vi "Transient SA.vi"() -> ()   [LabVIEW 2015]
uses:
  <vilib>/Platform/TimedLoop/XDataNode/timing_clust.ctl
  <vilib>/Platform/TimedLoop/XDataNode/nitl_modes.ctl
  <vilib>/Platform/TimedLoop/XDataNode/wakeup.ctl
  <vilib>/DAQmx/read.llb/DAQmx Read (Analog DBL 1Chan 1Samp).vi
  <vilib>/DAQmx/read.llb/DAQmx Read (Analog 1D DBL NChan 1Samp).vi
  <vilib>/DAQmx/create/channels.llb/DAQmx Create Channel (AI-Voltage-Basic).vi
  <vilib>/DAQmx/miscellaneous.llb/DAQmx Fill In Error Info.vi
  <vilib>/Platform/TimedLoop/XDataNode/XDataNode.xnode
  Program Files/neMESYS_SDK/neMESYS LabVIEW Kit/neMESYS LabVIEW Integration Kit.lvlib
  <vilib>/Platform/TimedLoop/XDataNode/XDNodeRunTimeDep.lvlib
  Conor/Temp CN7500/Omega CN7500/Omega CN7500.lvlib
panel:
  out "Iteration Number":dbl
  in  "Ramp Temp":bool
  in  "Temp Decrease per Minute":dbl
  in  "Start Temp":dbl
  in  "Minutes at Start Conditions":dbl
  in  "Ramp Flow":bool
  in  "Flow Decrease per Minute":dbl
  in  "Start Flowrate":dbl
  in  "Flowrate 4":dbl
  in  "Flowrate 3":dbl
  in  "Flowrate 2":dbl
  in  "Flowrate 1":dbl
  in  "Temp Set Point":dbl
  out "Liquid Inlet Pressure (bar g)":dbl
  in  "Liquid P sensor Terminal Configuration":i32(ring)=-1 items=["default"=-1, "RSE"=10083, "NRSE"=10078, "Differential"=10106, "Pseudodifferential"=12529]
  in  "Liquid P sensor Physical Channel":tag="Dev1/ai0"
  in  "Safety or Emergency Syringe Control":bool
  out "Total Flowrate (uL/min)":dbl
  out "Gas Back Pressure (barg)":dbl
  in  "Shut down in empty?\nLeft off, right on":bool
  in  "Clear":bool
  out "Safety Shut Down Pressure (barg)":dbl
  out "Calculated Pressure":dbl[](graph)
  out "Safety Shut Down Temp":dbl
  out "Actual Temp (oC)":dbl
  out "Temperature":dynamicdata(graph)
  out "Temp Set Point (oC)":dbl
  in  "Stop everything":bool
  in  "Refill 4":bool
  in  "Refill 3":bool
  in  "Refill 2":bool
  in  "Refill 1":bool
  in  "Empty 4":bool
  in  "Empty 3":bool
  in  "Empty 2":bool
  in  "Empty 1":bool
  in  "Calibrate 4":bool
  in  "Calibrate 3":bool
  in  "Calibrate 2":bool
  in  "Calibrate 1":bool
  in  "Stop Dose 4":bool
  in  "Stop Dose 3":bool
  in  "Stop Dose 2":bool
  in  "Stop Dose 1":bool
  out "Syringe Level 4":dbl(slide) scale=0.0..5500.0
  out "Syringe Level 3":dbl(slide) scale=0.0..5500.0
  out "Syringe Level 2":dbl(slide) scale=0.0..5500.0
  out "Syringe Level 1":dbl(slide) scale=0.0..5500.0
  out "Flowrate 4 Ethanol":dbl
  out "Flowrate 3 Acid":dbl
  out "Flowrate 2 High":dbl
  out "Flowrate 1 Low":dbl
  # "Safety (start and end)"
  # "Current Conditions"
  # "(uL/min)"
  # "Coerced to nearest possible"
  # "If either ramps are off you need to manually enter the constant flowrate or temperature in the \nbottom sections"
  # "This code just uses 2 syringes\nThe ones at the right hand side"
  # "Emergency Syringe Control Below"
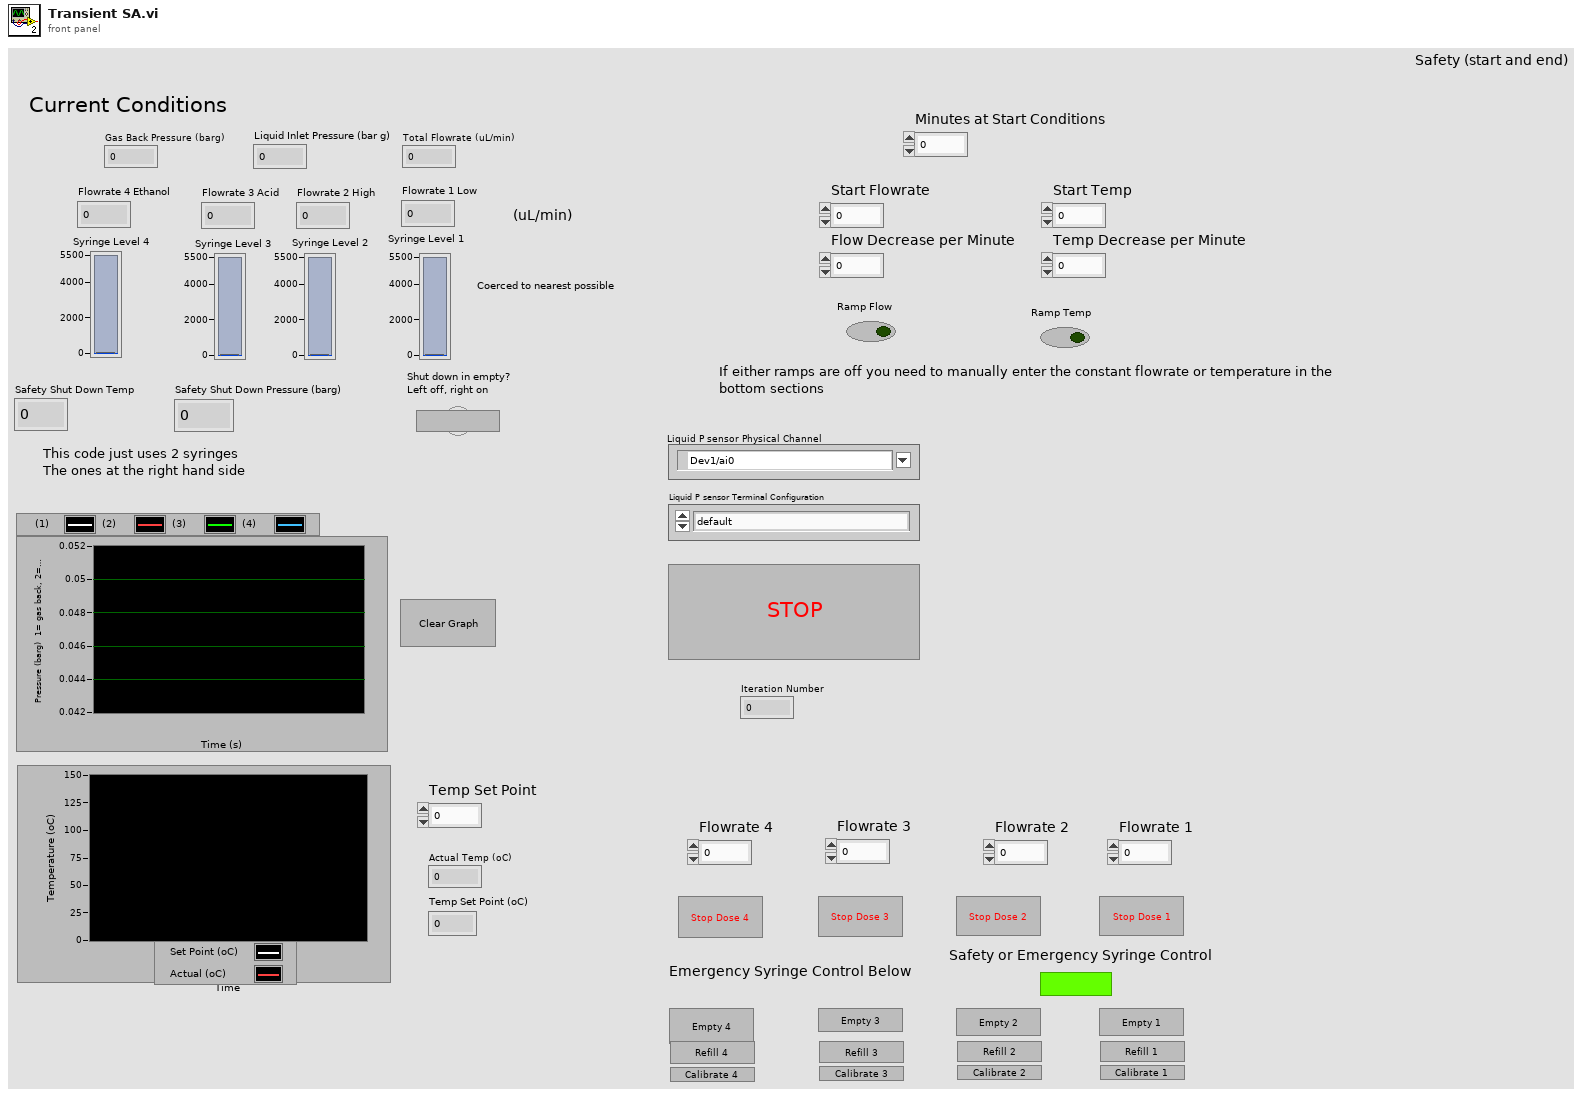
[diagram p1: front panel]
types:
  T1 = typedef "XDNodeRunTimeDep.lvlib/timing_clust.ctl" = cluster{"Expected End [f-1]":u64, "Actual End [f-1]":u64, "Finished Late? [f-1]":bool, "Expected End [i-1]":u64, "Actual End [i-1]":u64, "Finished Late? [i-1]":bool, "Expected Start [i]":u64, "Actual Start [i]":u64, "Expected Start [f]":u64, "Actual Start [f]":u64, "Source Name":string, "Structure Name":string, "Period":i64, "Deadline":i64, "Offset":i64, "Start":i64, "Priority":i32, "Timeout":i32, "Mode":T2, "Wakeup Reason":T3, "Error":errorcluster, "Source Type":string, "Secondary Source Type":string, "Global End Time":u64, "Global Start Time":u64, "Frame Duration":u64, "Iteration Duration":u64, "Assigned CPU":i32, "I/O Scan Engine Mode":u32}
  T2 = typedef "XDNodeRunTimeDep.lvlib/nitl_modes.ctl" = enum32{"No Change", "Process missed periods, maintain original phase", "Discard missed periods, maintain original phase", "Process missed periods, ignore original phase", "Discard missed periods, ignore original phase"}
  T3 = typedef "XDNodeRunTimeDep.lvlib/wakeup.ctl" = enum32{"Normal", "Aborted", "Asynchronous wakeup", "Timing source error", "Timed loop error", "Timeout"}
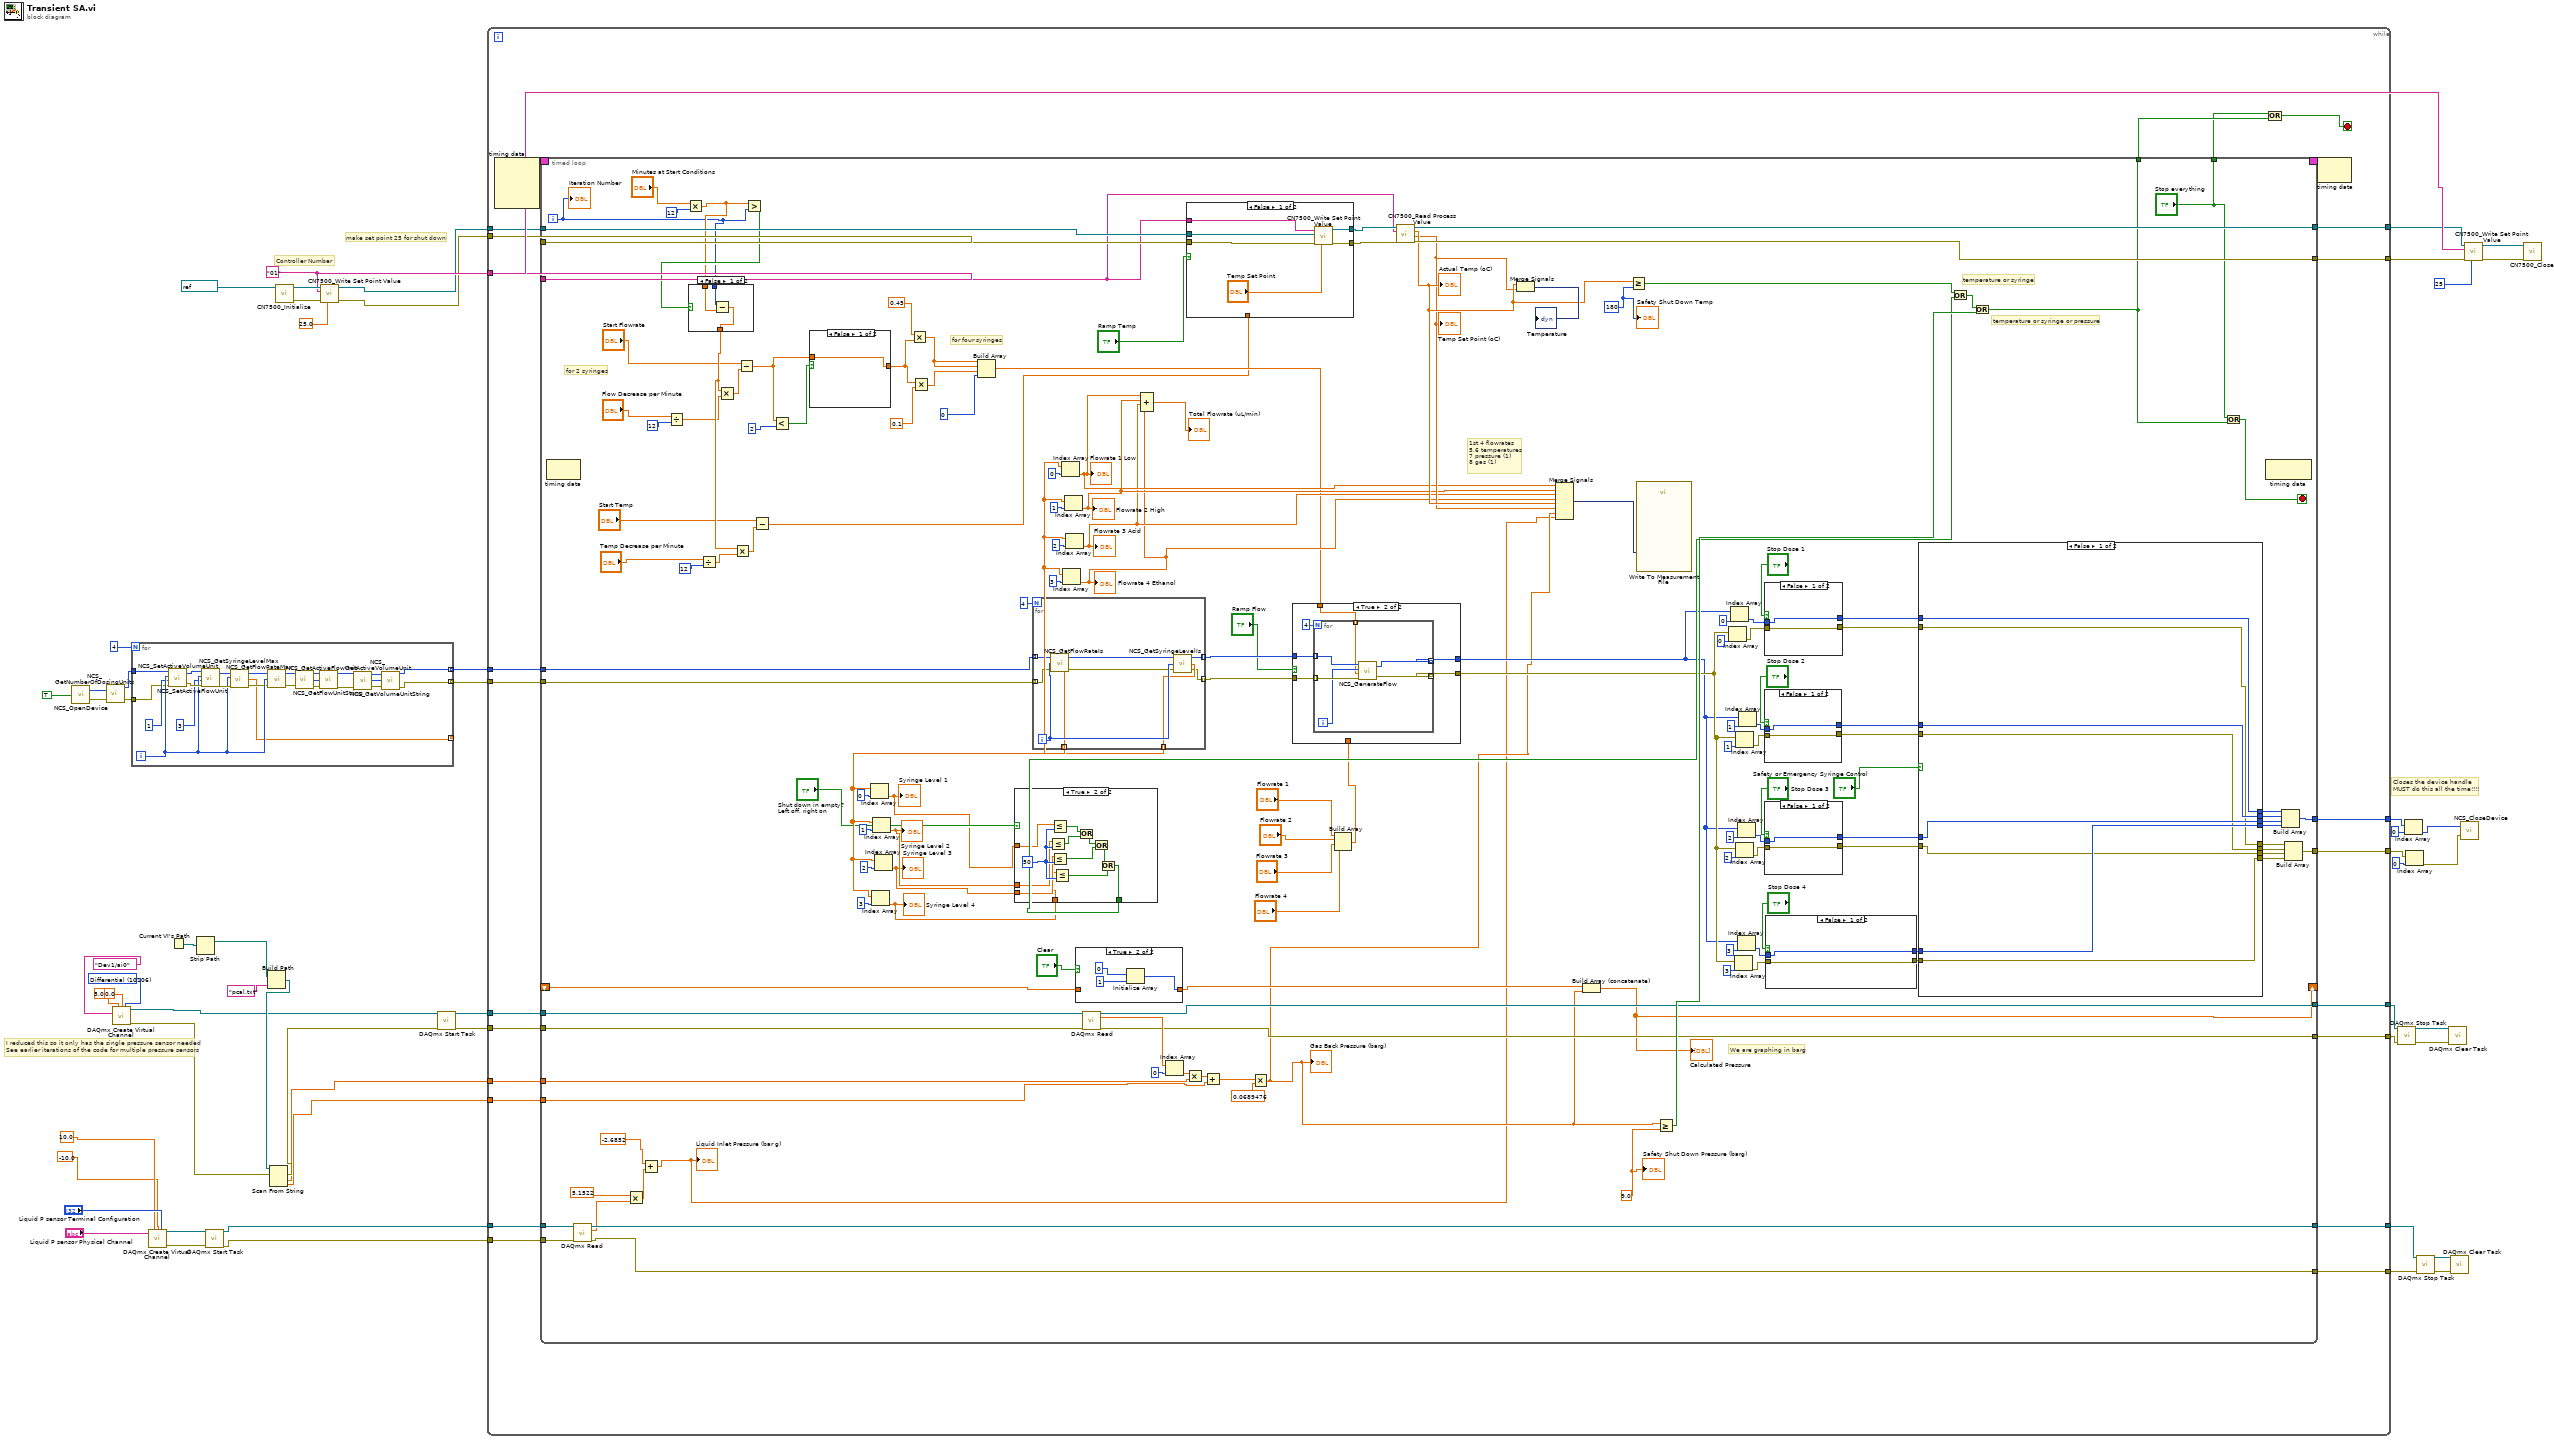
[diagram p0: block diagram]
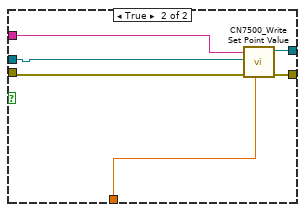
[diagram p2: hidden frame]
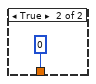
[diagram p3: hidden frame]
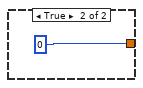
[diagram p4: hidden frame]
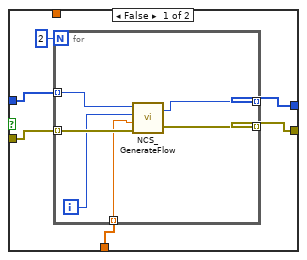
[diagram p5: hidden frame]
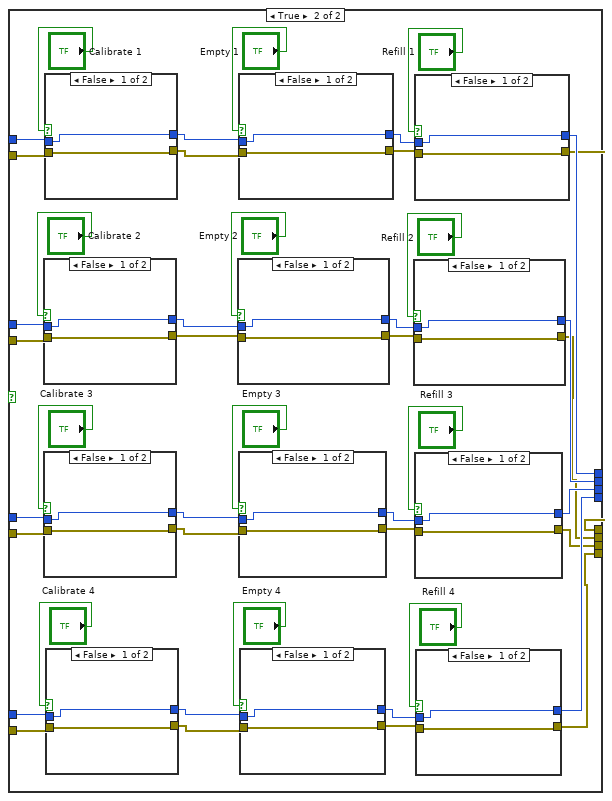
[diagram p6: hidden frame]
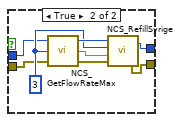
[diagram p7: hidden frame]
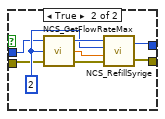
[diagram p8: hidden frame]
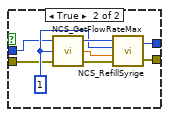
[diagram p9: hidden frame]
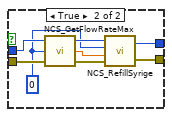
[diagram p10: hidden frame]
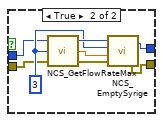
[diagram p11: hidden frame]
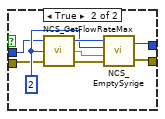
[diagram p12: hidden frame]
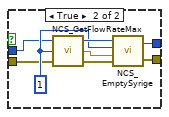
[diagram p13: hidden frame]
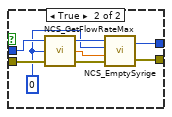
[diagram p14: hidden frame]
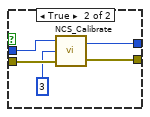
[diagram p15: hidden frame]
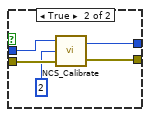
[diagram p16: hidden frame]
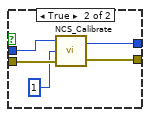
[diagram p17: hidden frame]
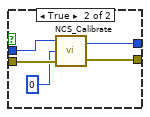
[diagram p18: hidden frame]
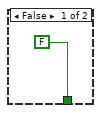
[diagram p19: hidden frame]
diagram:
  w29 = 10106 items=["default"=-1, "RSE"=10083, "NRSE"=10078, "Differential"=10106, "Pseudodifferential"=12529] ("input terminal configuration")
  w36 = "01" ("Controller Number")
  # "I reduced this so it only has the single pressure sensor needed\nSee earlier iterations of the code for multiple pressure sensors"
  # "make set point 25 for shut down"
  # "Controller Number"
  # "Closes the device handle \nMUST do this all the time!!!!"
  n1 = call "NCS_OpenDevice.vi"("show status window"=TRUE) -> ("device handle"=w55:u32, "error out"=w54:errorcluster)
  n2 = call "NCS_GetNumberOfDosingUnits.vi"("device handle in"=w55, "error in (no error)"=w54) -> ("device handle out"=w52:u32, "error out"=w53:errorcluster)  [unwired: 1 out]
  n3 = call-poly <vilib>:"DAQmx Create Virtual Channel.vi"("maximum value"=5.0, "minimum value"=0.0, "input terminal configuration"=w29, "physical channels"=tag "Dev1/ai0") -> ("task out"=w13:refnum<k21>, "error out"=w14:errorcluster)  [unwired: 10 in]
  n4 = for {
    N: 4 -> [_]
    tunnel: [w61] -> w51 mode=indexing
    tunnel: [w60] -> w50 mode=indexing
    tunnel: [w74] -> _ mode=indexing
    tunnel: w53 -> [w59]
    tunnel: w52 -> [w58]
    i -> [w77]
    n5 = call "NCS_SetActiveVolumeUnit.vi"("error in (no error)"=w59, "active volume unit"=1, "dosingunit"=w77, "device handle in"=w58) -> ("error out"=w80:errorcluster, "device handle out"=w81:u32)
    n6 = call "NCS_SetActiveFlowUnit.vi"("error in (no error)"=w80, "active flow unit"=3, "dosingunit"=w77, "device handle in"=w81) -> ("error out"=w78:errorcluster, "device handle out"=w79:u32)
    n7 = call "NCS_GetSyringeLevelMax.vi"("error in (no error)"=w78, "dosingunit"=w77, "device handle in"=w79) -> ("error out"=w75:errorcluster, "syringe level max"=w74:dbl, "device handle out"=w76:u32)  [unwired: 1 out]
    n8 = call "NCS_GetFlowRateMax.vi"("error in (no error)"=w75, "dosingunit"=w77, "device handle in"=w76) -> ("error out"=w62:errorcluster, "device handle out"=w63:u32)  [unwired: 1 out]
    n9 = call "NCS_GetActiveFlowUnit.vi"("error in (no error)"=w62, "device handle in"=w63) -> ("error out"=w70:errorcluster, "active flow unit"=w69:u8, "device handle out"=w71:u32)  [unwired: 1 in]
    n10 = call "NCS_GetFlowUnitString.vi"("device handle in"=w71, "flow unit id"=w69, "error in (no error)"=w70) -> ("device handle out"=w66:u32, "error out"=w65:errorcluster)  [unwired: 2 out]
    n11 = call "NCS_GetActiveVolumeUnit.vi"("error in (no error)"=w65, "device handle in"=w66) -> ("error out"=w67:errorcluster, "active volume unit"=w68:u8, "device handle out"=w64:u32)  [unwired: 1 in]
    n12 = call "NCS_GetVolumeUnitString.vi"("device handle in"=w64, "volume unit id"=w68, "error in (no error)"=w67) -> ("device handle out"=w61:u32, "error out"=w60:errorcluster)  [unwired: 2 out]
  }
  n13 = call-poly <vilib>:"DAQmx Create Virtual Channel.vi"("maximum value"=10.0, "minimum value"=-10.0 ("maximum value"), "input terminal configuration"="Liquid P sensor Terminal Configuration", "physical channels"="Liquid P sensor Physical Channel") -> ("task out"=w9:refnum<k21>, "error out"=w10:errorcluster)  [unwired: 10 in]
  n14 = Current VI's Path() -> (path=w27:path)
  n15 = Strip Path(path=w27) -> (stripped path=w25:path)  [unwired: 1 out]
  n16 = call <vilib>:"DAQmx Start Task.vi"("task/channels in"=w9, "error in"=w10) -> ("task out"=w8:refnum<k21>, "error out"=w7:errorcluster)  [unwired: 12 in]
  n17 = Build Path(base path=w25, name or relative path="pcal.txt") -> (appended path=w26:path)
  n18 = Scan From String(w26, w14) -> (w23:errorcluster, output 1=w20:dbl, output 2=w19:dbl)  [unwired: 3 in, 1 out]
  n19 = call "CN7500_Initialize.vi"("VISA resource name"=refnum<visa-resource-name> "COM8") -> ("error out"=w42:errorcluster, "VISA resource name out"=w43:refnum<visa-resource-name>)  [unwired: 9 in]
  n20 = call "CN7500_Write Set Point Value.vi"("Target Set Point Value"=25.0, "error in (no error)"=w42, "Controller Number"=w36, "VISA In"=w43) -> ("error out"=w34:errorcluster, "VISA Out"=w35:refnum<visa-resource-name>)  [unwired: 6 in]
  n21 = call <vilib>:"DAQmx Start Task.vi"("task/channels in"=w13, "error in"=w23) -> ("task out"=w22:refnum<k21>, "error out"=w21:errorcluster)  [unwired: 12 in]
  n22 = while {
    tunnel: w51 -> [w105]
    tunnel: w50 -> [w104]
    tunnel: [w103] -> w45
    tunnel: [w102] -> w44
    tunnel: w36 -> [w99]
    tunnel: w35 -> [w98]
    tunnel: w34 -> [w97]
    tunnel: [w96] -> w33
    tunnel: [w95] -> w32
    tunnel: w22 -> [w93]
    tunnel: w21 -> [w92]
    tunnel: w20 -> [w91]
    tunnel: w19 -> [w90]
    tunnel: [w89] -> w16
    tunnel: [w88] -> w15
    tunnel: w8 -> [w85]
    tunnel: w7 -> [w84]
    tunnel: [w83] -> w5
    tunnel: [w82] -> w3
    stop <- w87 stop-if-true
    n23 = node-c288() -> (w101:T1)  [unwired: 4 in]
    n24 = timed-loop {
      tunnel: w105 -> [w250]
      tunnel: w104 -> [w249]
      tunnel: [w200] -> w103
      tunnel: [w199] -> w102
      timing: w101 -> [_]
      timing-out: [_] -> w100
      tunnel: w99 -> [w193]
      tunnel: w98 -> [w197]
      tunnel: w97 -> [w196]
      tunnel: [w192] -> w96
      tunnel: [w191] -> w95
      tunnel: [w135] -> w94
      tunnel: w93 -> [w179]
      tunnel: w92 -> [w178]
      tunnel: w91 -> [w177]
      tunnel: w90 -> [w176]
      shift-right: [w156] -> _
      shift-left: _ -> [w169]
      tunnel: [w172] -> w89
      tunnel: [w171] -> w88
      tunnel: ["Stop everything"] -> w86
      tunnel: w85 -> [w155]
      tunnel: w84 -> [w154]
      tunnel: [w153] -> w83
      tunnel: [w152] -> w82
      i -> [w114]
      stop <- w167 stop-if-true
      w175 = 9.0 ("Safety Shut Down Pressure (barg)")
      w189 = 180
      # "for four syringes"
      # "for 2 syringes"
      # "1st 4 flowrates\n5,6 temperatures\n7 pressure (1)\n8 gas (1)"
      # "temperature or syringe or pressure"
      # "We are graphing in barg"
      # "temperature or syringe"
      n25 = node-c288() -> ()  [unwired: 1 in, 1 out]
      n26 = call-poly <vilib>:"DAQmx Read.vi"("task/channels in"=w155, "error in"=w154) -> ("task out"=w153:refnum<k21>, "data"=w148:dbl, "error out"=w152:errorcluster)  [unwired: 11 in]
      n27 = Multiply(x=5.1522, y=w148) -> (x*y=w151:dbl)
      n28 = Add(x=-2.6852, y=w151) -> (x+y=w146:dbl)
      "Liquid Inlet Pressure (bar g)" <- w146
      n29 = Divide(x="Flow Decrease per Minute", y=12) -> (x/y=w112:dbl)
      n30 = Multiply(x="Minutes at Start Conditions", y=12) -> (x*y=w123:dbl)
      n31 = Divide(x="Temp Decrease per Minute", y=12) -> (x/y=w119:dbl)
      n32 = Greater?(x=w123, y=w114) -> (0:w124:bool)
      n33 = case shown="False" w124 {
        tunnel: [w264 0] -> w118
        tunnel: w114 -> [w266 _]
        tunnel: w123 -> [w265 _]
        frame False {
          n34 = Subtract(x=w266, y=w265) -> (x-y=w264:dbl)
        }
        frame True {
        }
      }
      n35 = Multiply(x=w118, y=w112) -> (x*y=w132:dbl)
      n36 = Multiply(x=w118, y=w119) -> (x*y=w120:dbl)
      n37 = Subtract(x="Start Flowrate", y=w132) -> (x-y=w127:dbl)
      n38 = Subtract(x="Start Temp", y=w120) -> (x-y=w115:dbl)
      n39 = Less?(x=w127, y=2) -> (x < y?=w128:bool)
      n40 = case shown="False" w128 {
        tunnel: [w268 0] -> w108
        tunnel: w127 -> [w268 _]
        frame False {
        }
        frame True {
        }
      }
      n41 = Multiply(x=0.45, y=w108) -> (x*y=w107:dbl)
      n42 = Multiply(x=w108, y=0.1) -> (x*y=w106:dbl)
      n43 = Build Array(w107, w107, w106, 0) -> (w130:dbl[])
      n44 = for {
        N: 4 -> [_]
        tunnel: w250 -> [w509] mode=indexing
        tunnel: [w507] -> w244 mode=indexing
        tunnel: [w504] -> w239 mode=indexing
        tunnel: [w503] -> w238 mode=indexing
        tunnel: [w502] -> w237 mode=indexing
        tunnel: w249 -> [w501] mode=indexing
        i -> [w508]
        n45 = call "NCS_GetFlowRateIs.vi"("error in (no error)"=w501, "dosingunit"=w508, "device handle in"=w509) -> ("error out"=w505:errorcluster, "flowrate is"=w507:dbl, "device handle out"=w506:u32)
        n46 = call "NCS_GetSyringeLevelIs.vi"("error in (no error)"=w505, "dosingunit"=w508, "device handle in"=w506) -> ("error out"=w502:errorcluster, "syringe level is"=w504:dbl, "device handle out"=w503:u32)
      }
      n47 = Index Array(array=w239, index=0) -> (element=w164:dbl)
      "Syringe Level 1" <- w164
      n48 = Index Array(array=w239, index=3) -> (element=w161:dbl)
      "Syringe Level 4" <- w161
      n49 = Index Array(array=w239, index=1) -> (element=w163:dbl)
      "Syringe Level 2" <- w163
      n50 = Index Array(array=w239, index=2) -> (element=w162:dbl)
      "Syringe Level 3" <- w162
      n51 = case shown="True" "Shut down in empty?\nLeft off, right on" {
        tunnel: [FALSE w459] -> w165
        tunnel: w164 -> [_ w458]
        tunnel: w163 -> [_ w457]
        tunnel: w162 -> [_ w456]
        tunnel: w161 -> [_ w455]
        frame False {
        }
        frame True {
          w460 = 50
          n52 = Less Or Equal?(x=w457, y=w460) -> (x <= y?=w466:bool)
          n53 = Less Or Equal?(x=w458, y=w460) -> (x <= y?=w461:bool)
          n54 = Less Or Equal?(x=w456, y=w460) -> (x <= y?=w464:bool)
          n55 = Less Or Equal?(x=w455, y=w460) -> (x <= y?=w462:bool)
          n56 = Or(x=w461, y=w466) -> (x .or. y?=w465:bool)
          n57 = Or(x=w465, y=w464) -> (x .or. y?=w463:bool)
          n58 = Or(x=w463, y=w462) -> (x .or. y?=w459:bool)
        }
      }
      n59 = Index Array(array=w244, index=0) -> (element=w144:dbl)
      "Flowrate 1 Low" <- w144
      n60 = Index Array(array=w244, index=3) -> (element=w141:dbl)
      "Flowrate 4 Ethanol" <- w141
      n61 = Index Array(array=w244, index=1) -> (element=w143:dbl)
      "Flowrate 2 High" <- w143
      n62 = Index Array(array=w244, index=2) -> (element=w142:dbl)
      "Flowrate 3 Acid" <- w142
      n63 = case shown="True" "Clear" {
        tunnel: w169 -> [w467 _]
        tunnel: [w467 w468] -> w168
        frame False {
        }
        frame True {
          n64 = Initialize Array(0, 1) -> (w468:i32[])
        }
      }
      n65 = call-poly <vilib>:"DAQmx Read.vi"("task/channels in"=w179, "error in"=w178) -> ("task out"=w172:refnum<k21>, "data"=w184:dbl[], "error out"=w171:errorcluster)  [unwired: 11 in]
      n66 = Compound Arithmetic op=ADD(w144, w143, w142, w141) -> (→"Total Flowrate (uL/min)":dbl)
      n67 = Index Array(array=w184, index=0) -> (element=w182:dbl)
      n68 = Multiply(x=w182, y=w177) -> (x*y=w183:dbl)
      n69 = case shown="False" "Ramp Temp" {
        tunnel: w197 -> [w257 w262]
        tunnel: w196 -> [w256 w261]
        tunnel: [w255 w260] -> w195
        tunnel: [w254 w259] -> w194
        tunnel: w193 -> [w253 w263]
        tunnel: w115 -> [_ w258]
        frame False {
          n70 = call "CN7500_Write Set Point Value.vi"("Target Set Point Value"="Temp Set Point", "error in (no error)"=w256, "Controller Number"=w253, "VISA In"=w257) -> ("error out"=w254:errorcluster, "VISA Out"=w255:refnum<visa-resource-name>)  [unwired: 6 in]
        }
        frame True {
          n71 = call "CN7500_Write Set Point Value.vi"("Target Set Point Value"=w258, "error in (no error)"=w261, "Controller Number"=w263, "VISA In"=w262) -> ("error out"=w259:errorcluster, "VISA Out"=w260:refnum<visa-resource-name>)  [unwired: 6 in]
        }
      }
      n72 = Add(x=w183, y=w176) -> (x+y=w180:dbl)
      n73 = Multiply(x=w180, y=0.0689476) -> (x*y=w147:dbl)
      "Gas Back Pressure (barg)" <- w147
      n74 = Build Array("Flowrate 1", "Flowrate 2", "Flowrate 3", "Flowrate 4") -> (w136:dbl[])
      n75 = case shown="True" "Ramp Flow" {
        tunnel: w238 -> [w274 w287]
        tunnel: w237 -> [w273 w286]
        tunnel: [w271 w285] -> w159
        tunnel: [w270 w284] -> w158
        tunnel: w136 -> [w272 _]
        tunnel: w130 -> [_ w282]
        frame False {
          n76 = for {
            N: 2 -> [_]
            tunnel: w274 -> [w281] mode=indexing
            tunnel: w273 -> [w280] mode=indexing
            tunnel: [w279] -> w271 mode=indexing
            tunnel: [w278] -> w270 mode=indexing
            tunnel: w272 -> [w276] mode=indexing
            i -> [w277]
            n77 = call "NCS_GenerateFlow.vi"("error in (no error)"=w280, "flowrate"=w276, "dosingunit"=w277, "device handle in"=w281) -> ("error out"=w279:errorcluster, "device handle out"=w278:u32)
          }
        }
        frame True {
          n78 = for {
            N: 4 -> [_]
            tunnel: w287 -> [w293] mode=indexing
            tunnel: w286 -> [w292] mode=indexing
            tunnel: [w291] -> w285 mode=indexing
            tunnel: [w290] -> w284 mode=indexing
            tunnel: w282 -> [w288] mode=indexing
            i -> [w289]
            n79 = call "NCS_GenerateFlow.vi"("error in (no error)"=w292, "flowrate"=w288, "dosingunit"=w289, "device handle in"=w293) -> ("error out"=w291:errorcluster, "device handle out"=w290:u32)
          }
        }
      }
      n80 = call "CN7500_Read Process Value.vi"("error in (no error)"=w194, "Controller Number"=w193, "VISA In"=w195) -> ("error out"=w192:errorcluster, "Set Point Value"=w186:dbl, "Process Value"=w187:dbl, "VISA Out"=w191:refnum<visa-resource-name>)  [unwired: 5 in]
      "Temp Set Point (oC)" <- w186
      "Actual Temp (oC)" <- w187
      n81 = Merge Signals(w187, w186) -> (→"Temperature":dynamicdata)
      n82 = Merge Signals(w144, w143, w142, w141, w187, w186, w147, w146) -> (w198:dynamicdata)
      n83 = Build Array (concatenate)(w168, w147) -> (w156:dbl[])
      "Calculated Pressure" <- w156
      n84 = Greater Or Equal?(x=w187, y=w189) -> (x >= y?=w188:bool)
      n85 = call "Write To Measurement File"("Signals"=w198) -> ()  [unwired: 16 in, 3 out]
      n86 = Greater Or Equal?(x=w147, y=w175) -> (x >= y?=w173:bool)
      n87 = Index Array(array=w159, index=0) -> (element=w227:errorcluster)
      n88 = Index Array(array=w158, index=0) -> (element=w228:u32)
      n89 = Index Array(array=w159, index=3) -> (element=w217:errorcluster)
      n90 = Index Array(array=w159, index=2) -> (element=w219:errorcluster)
      n91 = Index Array(array=w159, index=1) -> (element=w221:errorcluster)
      n92 = Index Array(array=w158, index=3) -> (element=w218:u32)
      n93 = Index Array(array=w158, index=2) -> (element=w220:u32)
      n94 = Index Array(array=w158, index=1) -> (element=w222:u32)
      n95 = case shown="False" "Stop Dose 2" {
        tunnel: w222 -> [w488 w493]
        tunnel: w221 -> [w487 w492]
        tunnel: [w488 w491] -> w214
        tunnel: [w487 w490] -> w213
        frame False {
        }
        frame True {
          n96 = call "NCS_Stop.vi"("error in (no error)"=w492, "dosingunit"=1, "device handle in"=w493) -> ("error out"=w490:errorcluster, "device handle out"=w491:u32)
        }
      }
      n97 = case shown="False" "Stop Dose 1" {
        tunnel: w228 -> [w495 w500]
        tunnel: w227 -> [w494 w499]
        tunnel: [w495 w498] -> w216
        tunnel: [w494 w497] -> w215
        frame False {
        }
        frame True {
          n98 = call "NCS_Stop.vi"("error in (no error)"=w499, "dosingunit"=0, "device handle in"=w500) -> ("error out"=w497:errorcluster, "device handle out"=w498:u32)
        }
      }
      n99 = case shown="False" "Stop Dose 3" {
        tunnel: w220 -> [w481 w486]
        tunnel: w219 -> [w480 w485]
        tunnel: [w481 w484] -> w212
        tunnel: [w480 w483] -> w211
        frame False {
        }
        frame True {
          n100 = call "NCS_Stop.vi"("error in (no error)"=w485, "dosingunit"=2, "device handle in"=w486) -> ("error out"=w483:errorcluster, "device handle out"=w484:u32)
        }
      }
      n101 = case shown="False" "Stop Dose 4" {
        tunnel: w218 -> [w474 w479]
        tunnel: w217 -> [w473 w478]
        tunnel: [w474 w477] -> w210
        tunnel: [w473 w476] -> w209
        frame False {
        }
        frame True {
          n102 = call "NCS_Stop.vi"("error in (no error)"=w478, "dosingunit"=3, "device handle in"=w479) -> ("error out"=w476:errorcluster, "device handle out"=w477:u32)
        }
      }
      n103 = case shown="False" "Safety or Emergency Syringe Control" {
        tunnel: w216 -> [w301 w342]
        tunnel: w215 -> [w297 w341]
        tunnel: w214 -> [w300 w340]
        tunnel: w213 -> [w296 w339]
        tunnel: w212 -> [w299 w338]
        tunnel: w211 -> [w295 w337]
        tunnel: w210 -> [w298 w336]
        tunnel: w209 -> [w294 w335]
        tunnel: [w301 w312] -> w208
        tunnel: [w300 w311] -> w207
        tunnel: [w299 w310] -> w206
        tunnel: [w298 w309] -> w205
        tunnel: [w296 w308] -> w204
        tunnel: [w295 w307] -> w203
        tunnel: [w294 w306] -> w202
        tunnel: [w297 w302] -> w201
        frame False {
        }
        frame True {
          n104 = case shown="False" "Calibrate 2" {
            tunnel: w340 -> [w441 w446]
            tunnel: w339 -> [w440 w445]
            tunnel: [w441 w444] -> w329
            tunnel: [w440 w443] -> w328
            frame False {
            }
            frame True {
              n105 = call "NCS_Calibrate.vi"("error in (no error)"=w445, "dosingunit"=1, "device handle in"=w446) -> ("error out"=w443:errorcluster, "device handle out"=w444:u32)
            }
          }
          n106 = case shown="False" "Calibrate 3" {
            tunnel: w338 -> [w434 w439]
            tunnel: w337 -> [w433 w438]
            tunnel: [w434 w437] -> w327
            tunnel: [w433 w436] -> w326
            frame False {
            }
            frame True {
              n107 = call "NCS_Calibrate.vi"("error in (no error)"=w438, "dosingunit"=2, "device handle in"=w439) -> ("error out"=w436:errorcluster, "device handle out"=w437:u32)
            }
          }
          n108 = case shown="False" "Calibrate 1" {
            tunnel: w342 -> [w448 w453]
            tunnel: w341 -> [w447 w452]
            tunnel: [w448 w451] -> w331
            tunnel: [w447 w450] -> w330
            frame False {
            }
            frame True {
              n109 = call "NCS_Calibrate.vi"("error in (no error)"=w452, "dosingunit"=0, "device handle in"=w453) -> ("error out"=w450:errorcluster, "device handle out"=w451:u32)
            }
          }
          n110 = case shown="False" "Calibrate 4" {
            tunnel: w336 -> [w427 w432]
            tunnel: w335 -> [w426 w431]
            tunnel: [w427 w430] -> w325
            tunnel: [w426 w429] -> w324
            frame False {
            }
            frame True {
              n111 = call "NCS_Calibrate.vi"("error in (no error)"=w431, "dosingunit"=3, "device handle in"=w432) -> ("error out"=w429:errorcluster, "device handle out"=w430:u32)
            }
          }
          n112 = case shown="False" "Empty 2" {
            tunnel: w329 -> [w407 w411]
            tunnel: w328 -> [w406 w409]
            tunnel: [w407 w410] -> w315
            tunnel: [w406 w408] -> w316
            frame False {
            }
            frame True {
              w413 = 1
              n113 = call "NCS_GetFlowRateMax.vi"("error in (no error)"=w409, "dosingunit"=w413, "device handle in"=w411) -> ("error out"=w414:errorcluster, "flow rate max"=w412:dbl, "device handle out"=w415:u32)
              n114 = call "NCS_EmptySyrige.vi"("error in (no error)"=w414, "flowrate"=w412, "dosingunit"=w413, "device handle in"=w415) -> ("error out"=w408:errorcluster, "device handle out"=w410:u32)
            }
          }
          n115 = case shown="False" "Empty 1" {
            tunnel: w331 -> [w417 w425]
            tunnel: w330 -> [w416 w422]
            tunnel: [w417 w423] -> w313
            tunnel: [w416 w420] -> w314
            frame False {
            }
            frame True {
              w419 = 0
              n116 = call "NCS_GetFlowRateMax.vi"("error in (no error)"=w422, "dosingunit"=w419, "device handle in"=w425) -> ("error out"=w421:errorcluster, "flow rate max"=w418:dbl, "device handle out"=w424:u32)
              n117 = call "NCS_EmptySyrige.vi"("error in (no error)"=w421, "flowrate"=w418, "dosingunit"=w419, "device handle in"=w424) -> ("error out"=w420:errorcluster, "device handle out"=w423:u32)
            }
          }
          n118 = case shown="False" "Empty 3" {
            tunnel: w327 -> [w397 w398]
            tunnel: w326 -> [w396 w399]
            tunnel: [w397 w400] -> w317
            tunnel: [w396 w401] -> w318
            frame False {
            }
            frame True {
              w403 = 2
              n119 = call "NCS_GetFlowRateMax.vi"("error in (no error)"=w399, "dosingunit"=w403, "device handle in"=w398) -> ("error out"=w404:errorcluster, "flow rate max"=w402:dbl, "device handle out"=w405:u32)
              n120 = call "NCS_EmptySyrige.vi"("error in (no error)"=w404, "flowrate"=w402, "dosingunit"=w403, "device handle in"=w405) -> ("error out"=w401:errorcluster, "device handle out"=w400:u32)
            }
          }
          n121 = case shown="False" "Empty 4" {
            tunnel: w325 -> [w387 w388]
            tunnel: w324 -> [w386 w389]
            tunnel: [w387 w391] -> w319
            tunnel: [w386 w390] -> w320
            frame False {
            }
            frame True {
              w393 = 3
              n122 = call "NCS_GetFlowRateMax.vi"("error in (no error)"=w389, "dosingunit"=w393, "device handle in"=w388) -> ("error out"=w394:errorcluster, "flow rate max"=w392:dbl, "device handle out"=w395:u32)
              n123 = call "NCS_EmptySyrige.vi"("error in (no error)"=w394, "flowrate"=w392, "dosingunit"=w393, "device handle in"=w395) -> ("error out"=w390:errorcluster, "device handle out"=w391:u32)
            }
          }
          n124 = case shown="False" "Refill 2" {
            tunnel: w315 -> [w367 w371]
            tunnel: w316 -> [w366 w369]
            tunnel: [w367 w370] -> w311
            tunnel: [w366 w368] -> w308
            frame False {
            }
            frame True {
              w373 = 1
              n125 = call "NCS_GetFlowRateMax.vi"("error in (no error)"=w369, "dosingunit"=w373, "device handle in"=w371) -> ("error out"=w374:errorcluster, "flow rate max"=w372:dbl, "device handle out"=w375:u32)
              n126 = call "NCS_RefillSyrige.vi"("error in (no error)"=w374, "flowrate"=w372, "dosingunit"=w373, "device handle in"=w375) -> ("error out"=w368:errorcluster, "device handle out"=w370:u32)
            }
          }
          n127 = case shown="False" "Refill 1" {
            tunnel: w313 -> [w377 w385]
            tunnel: w314 -> [w376 w382]
            tunnel: [w377 w383] -> w312
            tunnel: [w376 w380] -> w302
            frame False {
            }
            frame True {
              w379 = 0
              n128 = call "NCS_GetFlowRateMax.vi"("error in (no error)"=w382, "dosingunit"=w379, "device handle in"=w385) -> ("error out"=w381:errorcluster, "flow rate max"=w378:dbl, "device handle out"=w384:u32)
              n129 = call "NCS_RefillSyrige.vi"("error in (no error)"=w381, "flowrate"=w378, "dosingunit"=w379, "device handle in"=w384) -> ("error out"=w380:errorcluster, "device handle out"=w383:u32)
            }
          }
          n130 = case shown="False" "Refill 3" {
            tunnel: w317 -> [w357 w358]
            tunnel: w318 -> [w356 w359]
            tunnel: [w357 w360] -> w310
            tunnel: [w356 w361] -> w307
            frame False {
            }
            frame True {
              w363 = 2
              n131 = call "NCS_GetFlowRateMax.vi"("error in (no error)"=w359, "dosingunit"=w363, "device handle in"=w358) -> ("error out"=w364:errorcluster, "flow rate max"=w362:dbl, "device handle out"=w365:u32)
              n132 = call "NCS_RefillSyrige.vi"("error in (no error)"=w364, "flowrate"=w362, "dosingunit"=w363, "device handle in"=w365) -> ("error out"=w361:errorcluster, "device handle out"=w360:u32)
            }
          }
          n133 = case shown="False" "Refill 4" {
            tunnel: w319 -> [w347 w348]
            tunnel: w320 -> [w346 w349]
            tunnel: [w347 w351] -> w309
            tunnel: [w346 w350] -> w306
            frame False {
            }
            frame True {
              w353 = 3
              n134 = call "NCS_GetFlowRateMax.vi"("error in (no error)"=w349, "dosingunit"=w353, "device handle in"=w348) -> ("error out"=w354:errorcluster, "flow rate max"=w352:dbl, "device handle out"=w355:u32)
              n135 = call "NCS_RefillSyrige.vi"("error in (no error)"=w354, "flowrate"=w352, "dosingunit"=w353, "device handle in"=w355) -> ("error out"=w350:errorcluster, "device handle out"=w351:u32)
            }
          }
        }
      }
      n136 = Or(x=w188, y=w165) -> (x .or. y?=w174:bool)
      n137 = Or(x=w174, y=w173) -> (x .or. y?=w135:bool)
      n138 = Or(x="Stop everything", y=w135) -> (x .or. y?=w167:bool)
      n139 = node-c288() -> ()  [unwired: 1 in, 1 out]
      n140 = Build Array(w208, w207, w206, w205) -> (w200:u32[])
      n141 = Build Array(w201, w204, w203, w202) -> (w199:errorcluster[])
      "Safety Shut Down Temp" <- w189
      "Safety Shut Down Pressure (barg)" <- w175
      "Iteration Number" <- w114
    }
    n142 = Or(x=w86, y=w94) -> (x .or. y?=w87:bool)
    n143 = node-c288(w100) -> ()  [unwired: 1 out]
  }
  n144 = call <vilib>:"DAQmx Stop Task.vi"("task/channels in"=w16, "error in"=w15) -> ("task out"=w18:refnum<k21>, "error out"=w17:errorcluster)  [unwired: 12 in]
  n145 = Index Array(array=w45, index=0) -> (element=w47:u32)
  n146 = Index Array(array=w44, index=0) -> (element=w46:errorcluster)
  n147 = call <vilib>:"DAQmx Stop Task.vi"("task/channels in"=w5, "error in"=w3) -> ("task out"=w4:refnum<k21>, "error out"=w6:errorcluster)  [unwired: 12 in]
  n148 = call <vilib>:"DAQmx Clear Task.vi"("task in"=w18, "error in"=w17) -> ()  [unwired: 13 in, 1 out]
  n149 = call <vilib>:"DAQmx Clear Task.vi"("task in"=w4, "error in"=w6) -> ()  [unwired: 13 in, 1 out]
  n150 = call "NCS_CloseDevice.vi"("error in (no error)"=w46, "device handle"=w47) -> ()  [unwired: 1 out]
  n151 = call "CN7500_Write Set Point Value.vi"("Target Set Point Value"=25, "error in (no error)"=w33, "Controller Number"=w36, "VISA In"=w32) -> ("error out"=w38:errorcluster, "VISA Out"=w39:refnum<visa-resource-name>)  [unwired: 6 in]
  n152 = call "CN7500_Close.vi"("error in (no error)"=w38, "VISA resource name"=w39) -> ()  [unwired: 9 in, 1 out]
